vi "Telnet_Challenge.vi"(8 "error in (no error)":errorcluster, 11 "connection ID in":refnum<k5>) -> (0 "error out":errorcluster, 2 "Challenge status":string, 3 "connection ID out":refnum<k5>)   [LabVIEW 2018]
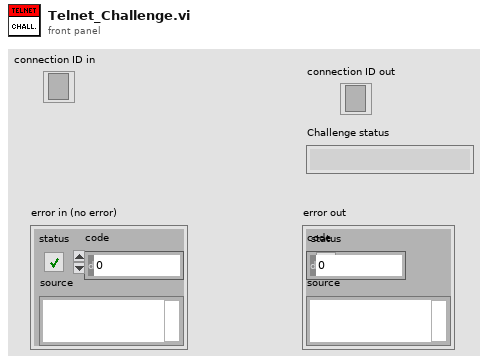
[diagram p1: front panel]
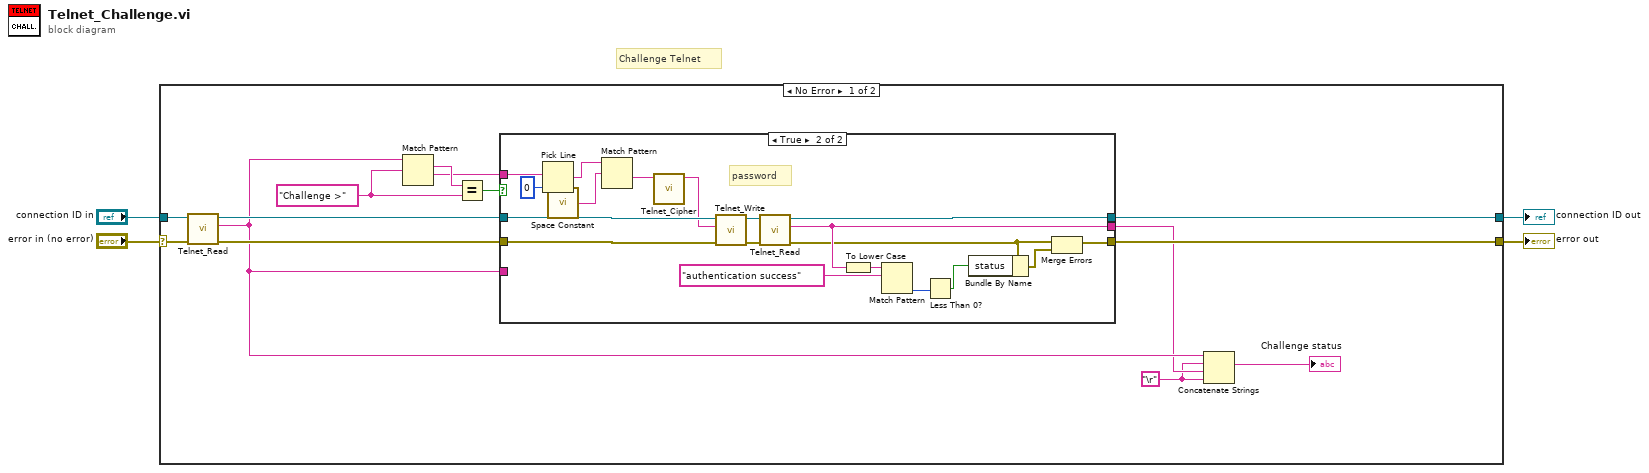
[diagram p0: block diagram]
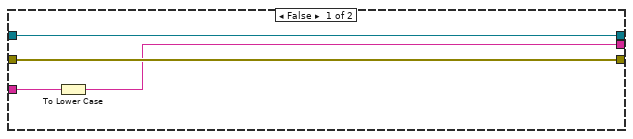
[diagram p2: hidden frame]
diagram:
  # "Challenge Telnet"
  n1 = case shown="No Error" "error in (no error)" {
    selector: "error in (no error)" -> [w11 w42]
    tunnel: [w14 w43] -> w4
    tunnel: [w13 w42] -> w3
    tunnel: "connection ID in" -> [w12 w43]
    frame No Error {
      w6 = "\r"
      w18 = "Challenge >" ("regular expression")
      n2 = call "Telnet_Read.vi"("error in (no error)"=w11, "connection ID In"=w12) -> ("error out"=w10:errorcluster, "string out"=w8:string, "connection ID out"=w9:refnum<k5>)  [unwired: 7 in]
      n3 = Match Pattern(string=w8, regular expression=w18) -> (match substring=w17:string, after substring=w15:string)  [unwired: 1 in, 2 out]
      n4 = Equal?(x=w17, y=w18) -> (x = y?=w16:bool)
      n5 = case shown="True" w16 {
        tunnel: w15 -> [_ w40]
        tunnel: w9 -> [w22 w30]
        tunnel: w10 -> [w21 w28]
        tunnel: [w22 w24] -> w14
        tunnel: [w21 w34] -> w13
        tunnel: [w19 w25] -> w7
        tunnel: w8 -> [w20 _]
        frame False {
          n6 = To Lower Case(string=w20) -> (all lower case string=w19:string)
        }
        frame True {
          # "password"
          n7 = Pick Line(multi-line string=w40, line index=0) -> (output string=w39:string)  [unwired: 1 in]
          n8 = call "Space Constant.vi"() -> ("String"=w38:string)
          n9 = Match Pattern(string=w39, regular expression=w38) -> (after substring=w31:string)  [unwired: 1 in, 3 out]
          n10 = call "Telnet_Cipher.vi"("Challenge"=w31) -> ("Response"=w29:string)  [unwired: 10 in]
          n11 = call "Telnet_Write.vi"("error in (no error)"=w28, "Write Telnet Command"=w29, "Telnet address ref"=w30) -> ("error out"=w27:errorcluster, "connection ID out"=w26:refnum<k5>)  [unwired: 7 in]
          n12 = call "Telnet_Read.vi"("error in (no error)"=w27, "connection ID In"=w26) -> ("error out"=w23:errorcluster, "string out"=w25:string, "connection ID out"=w24:refnum<k5>)  [unwired: 7 in]
          n13 = To Lower Case(string=w25) -> (all lower case string=w37:string)
          n14 = Match Pattern(string=w37, regular expression="authentication success") -> (offset past match=w33:i32)  [unwired: 1 in, 3 out]
          n15 = Less Than 0?(x=w33) -> (x < 0?=w32:bool)
          n16 = Bundle By Name(cluster=w23, "status"=w32) -> (w35:errorcluster)
          n17 = Merge Errors(w23, w35) -> (w34:errorcluster)
        }
      }
      n18 = Concatenate Strings(w8, w6, w7, w6) -> (→"Challenge status":string)
    }
    frame Error {
    }
  }
  "connection ID out" <- w4
  "error out" <- w3
